vi "GOOP_CheckForDependencyViewer.vi"(11 "Configurations":string[](array[string])) -> (1 "PopUpMenu(IfExists)":T1[](array[typedef]), 2 "Dependency Viewer Path":path, 3 "Dependency Viewer Exists":bool)   [LabVIEW 2020]
uses:
  <resource>/Framework/Providers/API/mxLvMenuItem.ctl
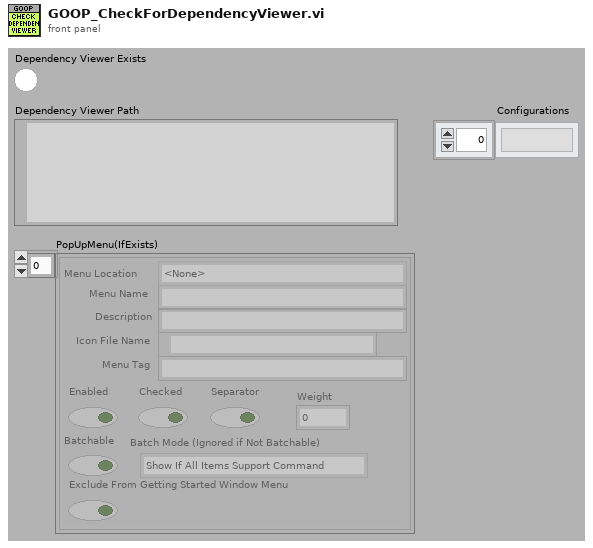
[diagram p1: front panel]
types:
  T1 = typedef "mxLvMenuItem.ctl" = cluster{"Menu Name":string, "Description":string, "Icon File Name":path, "Menu Tag":string, "Enabled":bool, "Checked":bool, "Separator":bool, "Batchable":bool, "Weight":i32, "Batch Mode (Ignored if Not Batchable)":enum32{"Show If All Items Support Command", "Show If Any Items Support Command"}, "Menu Location":enum32{"<None>", "Project", "Project / Build Specifications", "Tools", "Tools / Source Control", "Tools / Real-Time Module", "Help"}, "Exclude From Getting Started Window Menu":bool}
  T2 = typedef "GOOP_DependencySettings.ctl" = cluster{"KeepInMemory":bool, "Configurations":T3[]}
  T3 = typedef "DependencyChecker.lvlib/DependencyConfiguration.ctl" = cluster{"Name":string, "RemoveItemsBelongingToLibraries":bool, "RemoveEvenSubLibraries":bool, "FilterOptions":T4, "OnlyKeepCircularDepedencies":bool, "IgnoreLibrariesInCircularDependencies":bool}
  T4 = typedef "DependencyChecker.lvlib/FilterOptions.ctl" = cluster{"Ignore user.lib":bool, "Ignore vi.lib":bool, "Ignore instr.lib":bool, "FolderToIgnore":path[], "Ignore libraries":bool, "Ignore lvcasses":bool, "Ignore xnodes":bool, "Ignore xcontrols":bool, "Ignore Channel Classes":bool}
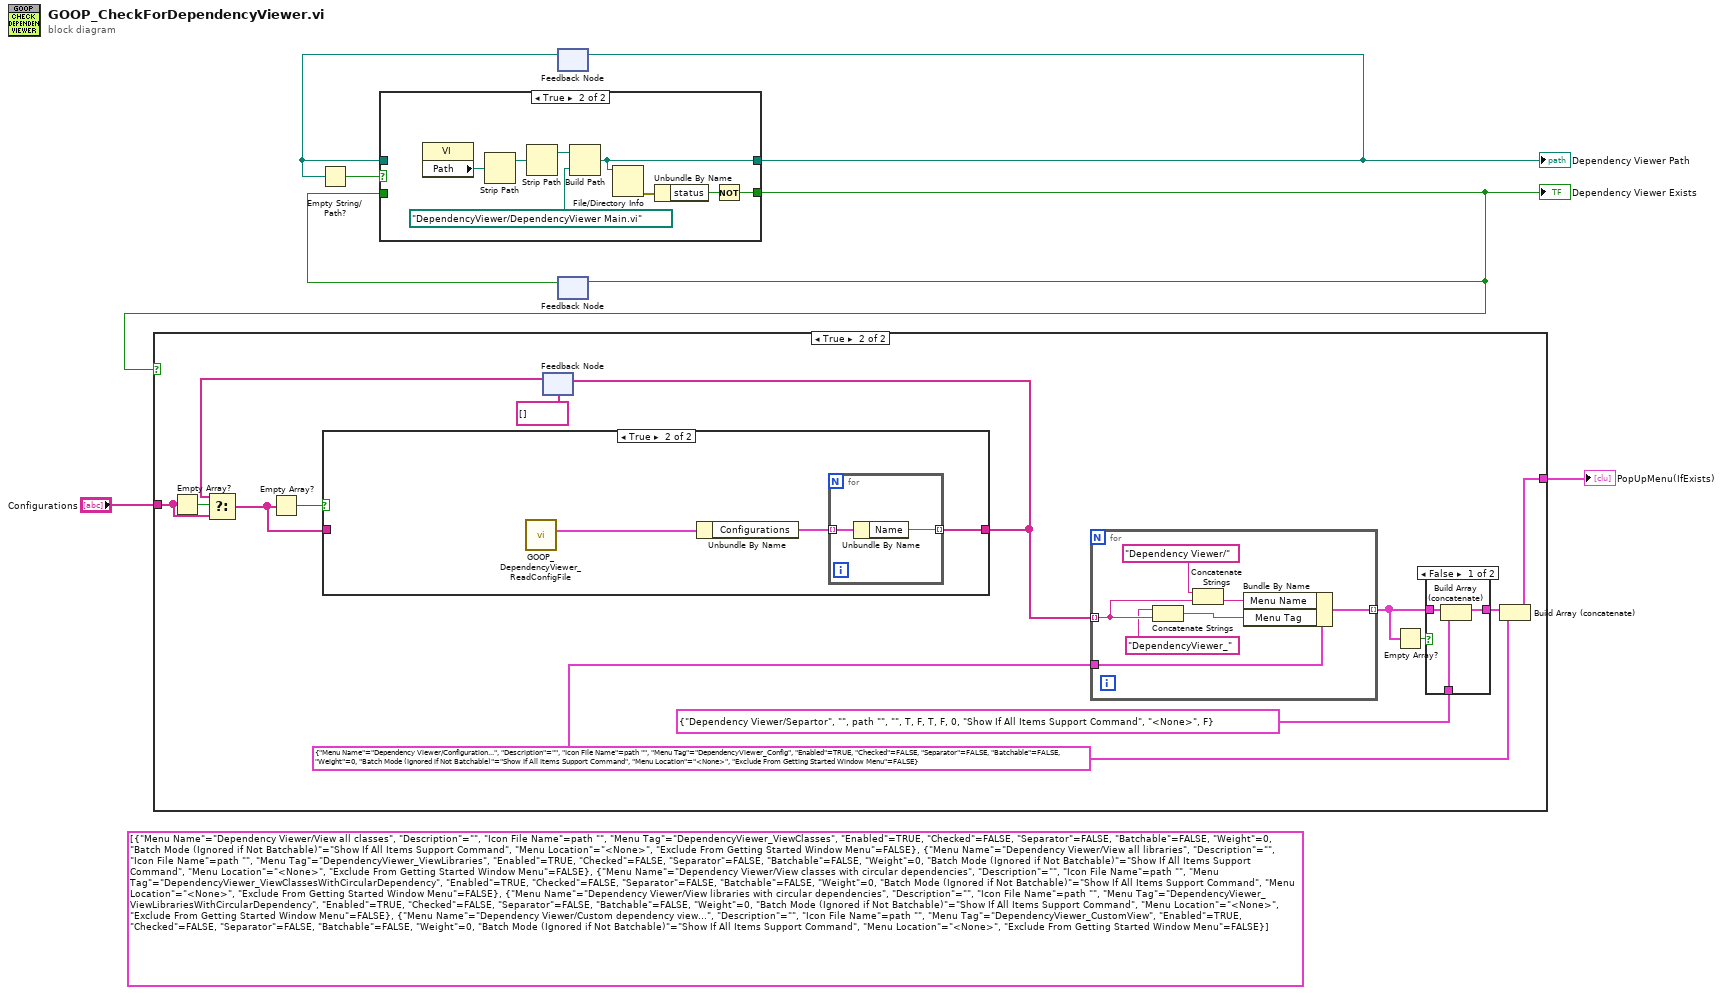
[diagram p0: block diagram]
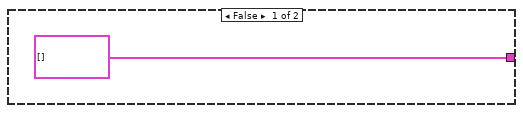
[diagram p2: hidden frame]
diagram:
  (unwired) T1[] [{"Menu Name"="Dependency Viewer/View all classes", "Description"="", "Icon File Name"=path "", "Menu Tag"="DependencyViewer_ViewClasses", "Enabled"=TRUE, "Checked"=FALSE, "Separator"=FALSE, "Batchable"=FALSE, "Weight"=0, "Batch Mode (Ignored if Not Batchable)"=enum."Show If All Items Support Command", "Menu Location"=enum."<None>", "Exclude From Getting Started Window Menu"=FALSE}, {"Menu Name"="Dependency Viewer/View all libraries", "Description"="", "Icon File Name"=path "", "Menu Tag"="DependencyViewer_ViewLibraries", "Enabled"=TRUE, "Checked"=FALSE, "Separator"=FALSE, "Batchable"=FALSE, "Weight"=0, "Batch Mode (Ignored if Not Batchable)"=enum."Show If All Items Support Command", "Menu Location"=enum."<None>", "Exclude From Getting Started Window Menu"=FALSE}, {"Menu Name"="Dependency Viewer/View classes with circular dependencies", "Description"="", "Icon File Name"=path "", "Menu Tag"="DependencyViewer_ViewClassesWithCircularDependency", "Enabled"=TRUE, "Checked"=FALSE, "Separator"=FALSE, "Batchable"=FALSE, "Weight"=0, "Batch Mode (Ignored if Not Batchable)"=enum."Show If All Items Support Command", "Menu Location"=enum."<None>", "Exclude From Getting Started Window Menu"=FALSE}, {"Menu Name"="Dependency Viewer/View libraries with circular dependencies", "Description"="", "Icon File Name"=path "", "Menu Tag"="DependencyViewer_ViewLibrariesWithCircularDependency", "Enabled"=TRUE, "Checked"=FALSE, "Separator"=FALSE, "Batchable"=FALSE, "Weight"=0, "Batch Mode (Ignored if Not Batchable)"=enum."Show If All Items Support Command", "Menu Location"=enum."<None>", "Exclude From Getting Started Window Menu"=FALSE}, {"Menu Name"="Dependency Viewer/Custom dependency view...", "Description"="", "Icon File Name"=path "", "Menu Tag"="DependencyViewer_CustomView", "Enabled"=TRUE, "Checked"=FALSE, "Separator"=FALSE, "Batchable"=FALSE, "Weight"=0, "Batch Mode (Ignored if Not Batchable)"=enum."Show If All Items Support Command", "Menu Location"=enum."<None>", "Exclude From Getting Started Window Menu"=FALSE}]
  n1 = feedback #1() -> (w4:path)  [unwired: 1 in]
  n2 = Empty String/Path?(string/path=w4) -> (empty?=w6:bool)
  n3 = feedback #2() -> (w5:bool)  [unwired: 1 in]
  n4 = case shown="True" w6 {
    tunnel: [w8 w11] -> w2
    tunnel: [w9 w10] -> w7
    tunnel: w5 -> [w8 _]
    tunnel: w4 -> [w9 _]
    frame False {
    }
    frame True {
      n5 = property class="VI"() -> ("Path"=w17:path)  [unwired: 2 in, 2 out]
      n6 = Strip Path(path=w17) -> (stripped path=w16:path)  [unwired: 1 out]
      n7 = Strip Path(path=w16) -> (stripped path=w15:path)  [unwired: 1 out]
      n8 = Build Path(base path=w15, name or relative path=path "DependencyViewer/DependencyViewer Main.vi") -> (appended path=w10:path)
      n9 = File/Directory Info(path=w10) -> (error out=w12:errorcluster)  [unwired: 1 in, 6 out]
      n10 = Unbundle By Name(w12) -> ("status"=w13:bool)
      n11 = Not(x=w13) -> (.not. x?=w11:bool)
    }
  }
  "Dependency Viewer Path" <- w7
  "Dependency Viewer Exists" <- w2
  n12 = case shown="True" w2 {
    tunnel: "Configurations" -> [_ w19]
    tunnel: [T1[] [] ("f") w20] -> w1
    frame False {
    }
    frame True {
      w21 = T1 {"Menu Name"="Dependency Viewer/Configuration...", "Description"="", "Icon File Name"=path "", "Menu Tag"="DependencyViewer_Config", "Enabled"=TRUE, "Checked"=FALSE, "Separator"=FALSE, "Batchable"=FALSE, "Weight"=0, "Batch Mode (Ignored if Not Batchable)"=enum."Show If All Items Support Command", "Menu Location"=enum."<None>", "Exclude From Getting Started Window Menu"=FALSE} ("Menu Item")
      n13 = Empty Array?(array=w19) -> (empty?=w30:bool)
      n14 = feedback #3(string[] [] ("Configurations")) -> (w29:string[])
      n15 = Select(t=w29, s=w30, f=w19) -> (s? t:f=w27:string[])
      n16 = Empty Array?(array=w27) -> (empty?=w28:bool)
      n17 = case shown="True" w28 {
        tunnel: [w43 w45] -> w26
        tunnel: w27 -> [w43 _]
        frame False {
        }
        frame True {
          n18 = call <resource>:"GOOP_DependencyViewer_ReadConfigFile.vi"() -> ("Config"=w44:T2)  [unwired: 11 in]
          n19 = Unbundle By Name(w44) -> ("Configurations"=w46:T3[])
          n20 = for {
            tunnel: w46 -> [w48] mode=indexing
            tunnel: [w47] -> w45 mode=indexing
            n21 = Unbundle By Name(w48) -> ("Name"=w47:string)
          }
        }
      }
      n22 = feedback-in #3(w26) -> ()
      n23 = for {
        tunnel: w21 -> [w42]
        tunnel: w26 -> [w39] mode=indexing
        tunnel: [w36] -> w25 mode=indexing
        n24 = Concatenate Strings("DependencyViewer_" ("string"), w39) -> (w38:string)
        n25 = Concatenate Strings("Dependency Viewer/" ("string"), w39) -> (w41:string)
        n26 = Bundle By Name(cluster=w42, "Menu Name"=w41, "Menu Tag"=w38) -> (w36:T1)
      }
      n27 = Empty Array?(array=w25) -> (empty?=w24:bool)
      n28 = case shown="False" w24 {
        tunnel: w25 -> [w34 w35]
        tunnel: T1 {"Menu Name"="Dependency Viewer/Separtor", "Description"="", "Icon File Name"=path "", "Menu Tag"="", "Enabled"=TRUE, "Checked"=FALSE, "Separator"=TRUE, "Batchable"=FALSE, "Weight"=0, "Batch Mode (Ignored if Not Batchable)"=enum."Show If All Items Support Command", "Menu Location"=enum."<None>", "Exclude From Getting Started Window Menu"=FALSE} ("Menu Item") -> [w33 _]
        tunnel: [w32 w35] -> w22
        frame False {
          n29 = Build Array (concatenate)(w34, w33) -> (w32:T1[])
        }
        frame True {
        }
      }
      n30 = Build Array (concatenate)(w22, w21) -> (w20:T1[])
    }
  }
  "PopUpMenu(IfExists)" <- w1
  n31 = feedback-in #1(w7) -> ()
  n32 = feedback-in #2(w2) -> ()
